vi "Logging module-status updater.vi"(8 "error in":errorcluster, 9 "Queue element":T1 {"Frame Size" items=["100X100"=100, "128X128"=128, "200X200"=200, "256X256"=256, "512X512"=512, "1024x1024"=1024, "2048x2048"=2048]; "Dwell time (us)" format="%#.6g"}, 11 "Message Queues":T5) -> (0 "error out":errorcluster)   [LabVIEW 2013]
uses:
  User Interface/Queue/Message Queue/Typedefs/All Message Queues.ctl
  User Interface/Queue/Message Queue/Typedefs/Message Cluster.ctl
  Typedefs/Logging queue element.ctl
  Typedefs/Imaging Protocols enum.ctl
  Typedefs/Frame Size.ctl
  Typedefs/Acquired points count.ctl
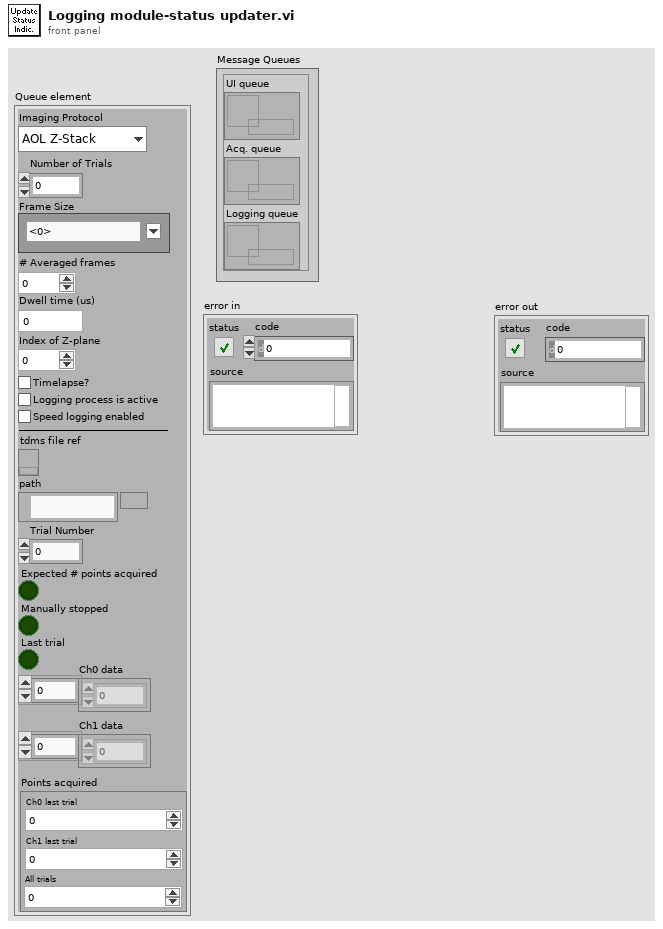
[diagram p1: front panel]
types:
  T1 = typedef "Logging queue element.ctl" = cluster{"Imaging Protocol":T2, "Number of Trials":u16, "Frame Size":T3, "# Averaged frames":u16, "Dwell time (us)":dbl, "Index of Z-plane":i32, "Timelapse?":bool, "Logging process is active":bool, "Speed logging enabled":bool, "tdms file ref":refnum<k34>, "path":path, "Trial Number":i32, "Expected # points acquired":bool, "Manually stopped":bool, "Ch0 data":u32[], "Ch1 data":u32[], "Last trial":bool, "Points acquired":T4}
  T2 = typedef "Imaging Protocols enum.ctl" = enum16{"AOL Z-Stack", "Motor Z Stack", "Functional Acquisition", "Single Plane Acquisition", "Volume Acquisition", "Live Imaging", "Live Plane Imaging", "Live Volume Imaging"}
  T3 = typedef "Frame Size.ctl" = u16
  T4 = typedef "Acquired points count.ctl" = cluster{"Ch0 last trial":u64, "Ch1 last trial":u64, "All trials":u64}
  T5 = typedef "All Message Queues.ctl" = cluster{"UI queue":refnum<queue>, "Acq. queue":refnum<queue>, "Logging queue":refnum<queue>}
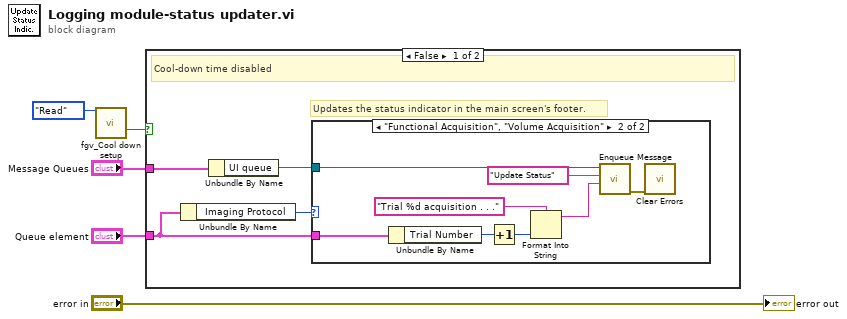
[diagram p0: block diagram]
diagram:
  n1 = call "fgv_Cool down setup.vi"("Function"=enum16{"Intialize", "Write", "Read", "Clear"}."Read") -> ("Enable cool-down time"=w1:bool)  [unwired: 12 in, 2 out]
  n2 = case shown="False" w1 {
    tunnel: "Message Queues" -> [w9 _]
    tunnel: "Queue element" -> [w7 _]
    frame False {
      # "Updates the status indicator in the main screen's footer."
      # "Cool-down time disabled"
      n3 = Unbundle By Name(w7) -> ("Imaging Protocol"=w6:T2)
      n4 = Unbundle By Name(w9) -> ("UI queue"=w8:refnum<queue>)
      n5 = case shown="\"Functional Acquisition\", \"Volume Acquisition\"" w6 {
        tunnel: w8 -> [_ w15]
        tunnel: w7 -> [_ w11]
        frame Default {
        }
        frame "Functional Acquisition", "Volume Acquisition" {
          n6 = Unbundle By Name(w11) -> ("Trial Number"=w12:i32)
          n7 = Increment(x=w12) -> (x+1=w10:i32)
          n8 = Format Into String(format string="Trial %d acquisition . . ." ("Acquiring and Logging..."), w10) -> (resulting string=w13:string)  [unwired: 2 in, 1 out]
          n9 = call "Enqueue Message.vi"("Message Data"=w13, "Message"="Update Status", "Queue"=w15) -> ("error out"=w16:errorcluster)  [unwired: 7 in, 1 out]
          n10 = call <vilib>:"Clear Errors.vi"("error in (no error)"=w16) -> ()  [unwired: 6 in, 1 out]
        }
      }
    }
    frame True {
      # "The status indicator is set by the \"Apply cool-down delay.vi\""
      # "Cool-down time enabled"
    }
  }
  "error out" <- "error in"
